vi "Write Serial Data.vi"(7 "error in":errorcluster, 9 "SerialData":refnum<class "Data.lvclass">[](array[class]), 10 "binFile":refnum<file>) -> (0 "error out":errorcluster, 3 "binFileOut":refnum<file>)   [LabVIEW 2012]
uses:
  Devices/Alicat/Data/MC/AlicatMCData.lvclass
  Controls/crd_data_enum.ctl
  Reusable/Data/Data.lvclass
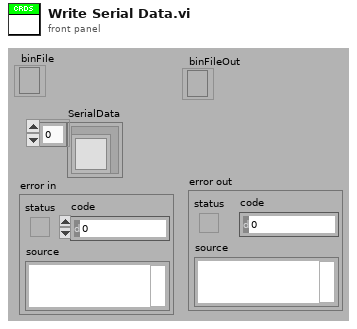
[diagram p1: front panel]
types:
  T1 = typedef "cPAS Library.lvlib/crd_data_enum.ctl" = enum8{"Time", "RHw", "TRH", "P", "Tmean", "RHsense", "TQ", "PQ", "Q", "Q0", "Qcal", "Qset", "extDilFac", "taucorr", "tau0corr", "stdevtau", "ext", "extCorr", "etau", "tau", "tau0", "Purge_Data", "NoData", "reserved", "Ttec", "Ang Exp", "Gamma", "filter", "fOverride", "notes", "max amp", "Tthermistor", "RhdilFac", "Psense", "TRHsense_bank", "RHsense_bank", "MFC_Data", "Thum", "ThumSP"}
  T2 = enum16{"big-endian, network order", "native, host order", "little-endian"}
  T3 = cluster{"P":sgl, "T":sgl, "Q":sgl, "Q0":sgl, "Qsp":sgl}
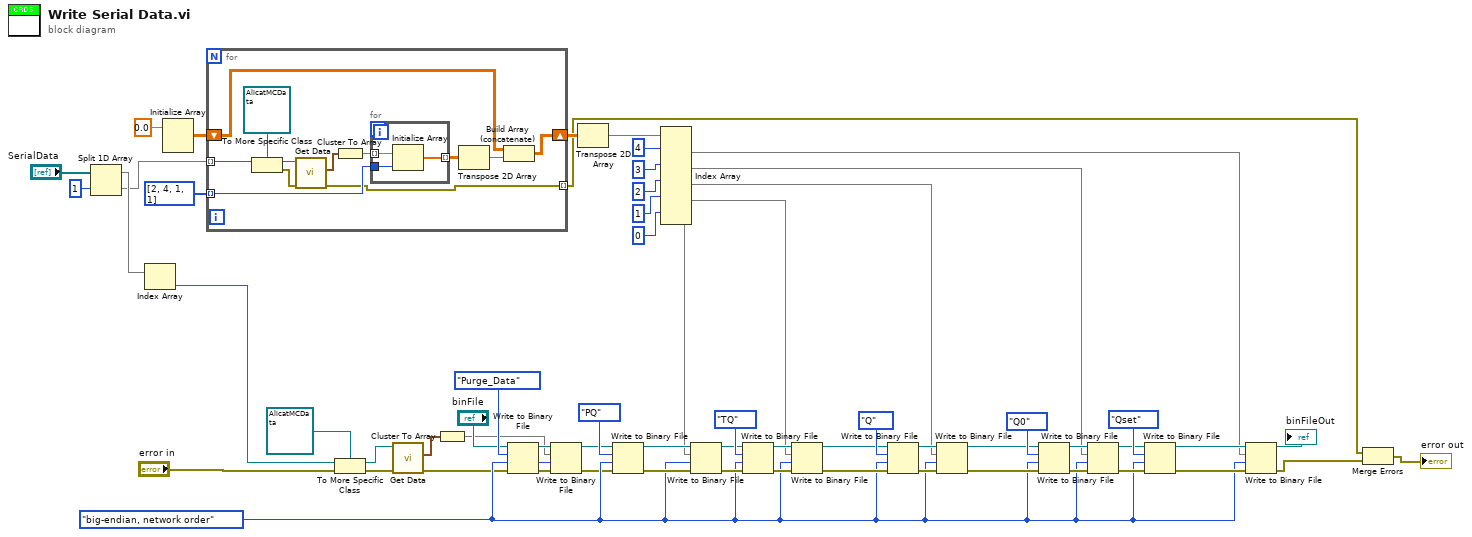
[diagram p0: block diagram]
diagram:
  w21 = T2."big-endian, network order" ("byte order (0:big-endian, network order)")
  n1 = Split 1D Array(array="SerialData", index=1) -> (first subarray=w7:refnum<class "Data.lvclass">[], second subarray=w4:refnum<class "Data.lvclass">[])
  n2 = Index Array(array=w7) -> (element=w5:refnum<class "Data.lvclass">)  [unwired: 1 in]
  n3 = Initialize Array(sgl 0.0 ("element")) -> (w53:sgl[][])  [unwired: 2 in]
  n4 = for {
    tunnel: w4 -> [w70] mode=indexing
    tunnel: i32[] [2, 4, 1, 1] -> [w67] mode=indexing
    shift-right: [w63] -> w52
    shift-left: w53 -> [w64]
    tunnel: [w62] -> w3 mode=indexing
    n5 = To More Specific Class(target class=refnum<class "AlicatMCData.lvclass"> refnum ("Alicat.lvlib:AlicatMCData.lvclass"), reference=w70) -> (specific class reference=w72:refnum<class "AlicatMCData.lvclass">, error out=w71:errorcluster)  [unwired: 1 in]
    n6 = call "Get Data.vi"("error in"=w71, "AlicatMData in"=w72) -> ("error out"=w62:errorcluster, "SystemData"=w69:T3)  [unwired: 7 in, 1 out]
    n7 = Cluster To Array(cluster=w69) -> (array=w68:sgl[])
    n8 = for {
      tunnel: w68 -> [w76] mode=indexing
      tunnel: w67 -> [w75]
      tunnel: [w74] -> w66 mode=indexing
      n9 = Initialize Array(w76, w75) -> (w74:sgl[])
    }
    n10 = Transpose 2D Array(2D array=w66) -> (transposed array=w65:sgl[][])
    n11 = Build Array (concatenate)(w64, w65) -> (w63:sgl[][])
  }
  n12 = To More Specific Class(target class=refnum<class "AlicatMCData.lvclass"> refnum ("Alicat.lvlib:AlicatMCData.lvclass"), reference=w5, error in="error in") -> (specific class reference=w60:refnum<class "AlicatMCData.lvclass">, error out=w61:errorcluster)
  n13 = call "Get Data.vi"("error in"=w61, "AlicatMData in"=w60) -> ("error out"=w14:errorcluster, "SystemData"=w13:T3)  [unwired: 7 in, 1 out]
  n14 = Cluster To Array(cluster=w13) -> (array=w12:sgl[])
  n15 = Write to Binary File(file (use dialog)="binFile", data=crd_data_enum."Purge_Data" ("CRD_Data_Enum"), error in=w14, 9:w21) -> (refnum out=w58:refnum<file>, error out=w15:errorcluster)  [unwired: 2 in, 1 out]
  n16 = Write to Binary File(file (use dialog)=w58, data=w12, error in=w15, 9:w21) -> (refnum out=w10:refnum<file>, error out=w9:errorcluster)  [unwired: 2 in, 1 out]
  n17 = Transpose 2D Array(2D array=w52) -> (transposed array=w51:sgl[][])
  n18 = Write to Binary File(file (use dialog)=w10, data=crd_data_enum."PQ" ("CRD_Data_Enum"), error in=w9, 9:w21) -> (refnum out=w44:refnum<file>, error out=w45:errorcluster)  [unwired: 2 in, 1 out]
  n19 = Index Array(array=w51, index (row) #1=4 ("index (row)"), index (row) #2=3 ("index (row)"), index (row) #3=2 ("index (row)"), index (row) #4=1 ("index (row)"), index (row) #5=0 ("index (row)")) -> (element #1=w17:sgl[], element #2=w18:sgl[], element #3=w32:sgl[], element #4=w19:sgl[], element #5=w20:sgl[])  [unwired: 5 in]
  n20 = Write to Binary File(file (use dialog)=w44, data=w20, error in=w45, 9:w21) -> (refnum out=w39:refnum<file>, error out=w38:errorcluster)  [unwired: 2 in, 1 out]
  n21 = Write to Binary File(file (use dialog)=w39, data=crd_data_enum."TQ" ("CRD_Data_Enum"), error in=w38, 9:w21) -> (refnum out=w42:refnum<file>, error out=w41:errorcluster)  [unwired: 2 in, 1 out]
  n22 = Write to Binary File(file (use dialog)=w42, data=w19, error in=w41, 9:w21) -> (refnum out=w34:refnum<file>, error out=w33:errorcluster)  [unwired: 2 in, 1 out]
  n23 = Write to Binary File(file (use dialog)=w34, data=crd_data_enum."Q" ("CRD_Data_Enum"), error in=w33, 9:w21) -> (refnum out=w36:refnum<file>, error out=w37:errorcluster)  [unwired: 2 in, 1 out]
  n24 = Write to Binary File(file (use dialog)=w36, data=w32, error in=w37, 9:w21) -> (refnum out=w28:refnum<file>, error out=w27:errorcluster)  [unwired: 2 in, 1 out]
  n25 = Write to Binary File(file (use dialog)=w28, data=crd_data_enum."Q0" ("CRD_Data_Enum"), error in=w27, 9:w21) -> (refnum out=w31:refnum<file>, error out=w30:errorcluster)  [unwired: 2 in, 1 out]
  n26 = Write to Binary File(file (use dialog)=w31, data=w18, error in=w30, 9:w21) -> (refnum out=w23:refnum<file>, error out=w22:errorcluster)  [unwired: 2 in, 1 out]
  n27 = Write to Binary File(file (use dialog)=w23, data=crd_data_enum."Qset" ("CRD_Data_Enum"), error in=w22, 9:w21) -> (refnum out=w25:refnum<file>, error out=w26:errorcluster)  [unwired: 2 in, 1 out]
  n28 = Write to Binary File(file (use dialog)=w25, data=w17, error in=w26, 9:w21) -> (refnum out=→"binFileOut":refnum<file>, error out=w2:errorcluster)  [unwired: 2 in, 1 out]
  n29 = Merge Errors(w3, w2) -> (→"error out":errorcluster)
